vi "Binary_Array_To_Decimal_Array.vi"(10 "Nmbr_of_datapoints":dbl=128.0, 11 "Array In":u8[](array[numeric])) -> (0 "HEXVAL":string, 1 "nV":dbl, 2 "Loop count":dbl, 3 "Array Out":dbl[](array[numeric]))   [LabVIEW 2012]
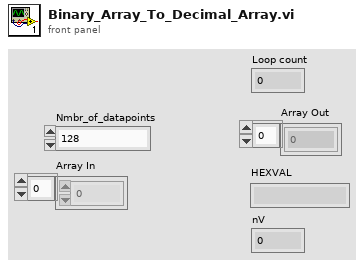
[diagram p1: front panel]
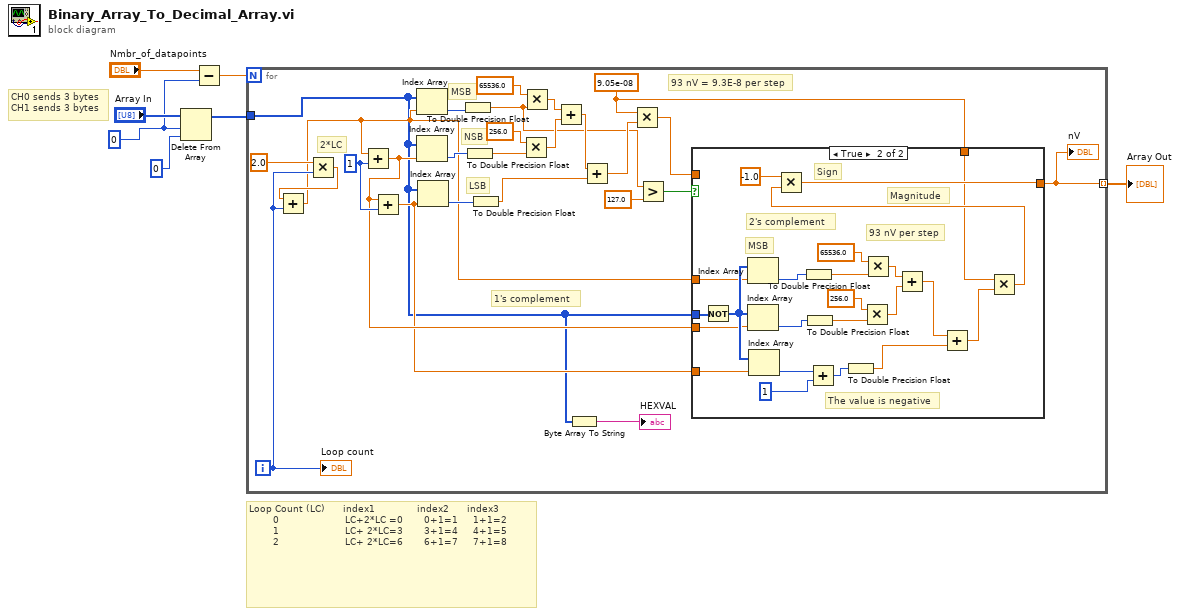
[diagram p0: block diagram]
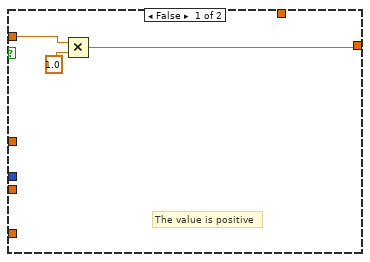
[diagram p2: hidden frame]
diagram:
  w3 = 0
  # "CH0 sends 3 bytes\nCH1 sends 3 bytes"
  # "Loop Count (LC)      index1              index2      index3      \n        0                      LC+2*LC =0       0+1=1     1+1=2\n        1                      LC+ 2*LC=3       3+1=4     4+1=5\n        2                      LC+ 2*LC=6       6+1=7     7+1=8"
  n1 = Delete From Array(array="Array In", length=w3, index=0) -> (array with subset deleted=w2:u8[])  [unwired: 1 out]
  n2 = Subtract(x="Nmbr_of_datapoints", y=w3) -> (x-y=w5:dbl)
  n3 = for {
    N: w5 -> [_]
    tunnel: w2 -> [w9]
    tunnel: [w8] -> w1 mode=indexing
    i -> [w15]
    w14 = 9.05e-08
    w25 = 1
    # "93 nV = 9.3E-8 per step"
    # "LSB"
    # "MSB"
    # "NSB"
    # "1's complement"
    # "2*LC"
    n4 = Multiply(x=2.0, y=w15) -> (x*y=w23:dbl)
    n5 = Add(x=w23, y=w15) -> (x+y=w13:dbl)
    n6 = Add(x=w13, y=w25) -> (x+y=w12:dbl)
    n7 = Add(x=w12, y=w25) -> (x+y=w11:dbl)
    n8 = Index Array(array=w9, index=w13) -> (element=w18:u8)
    n9 = Index Array(array=w9, index=w12) -> (element=w17:u8)
    n10 = Index Array(array=w9, index=w11) -> (element=w16:u8)
    n11 = To Double Precision Float(number=w18) -> (double precision float=w19:dbl)
    n12 = To Double Precision Float(number=w17) -> (double precision float=w31:dbl)
    n13 = To Double Precision Float(number=w16) -> (double precision float=w27:dbl)
    n14 = Multiply(x=256.0, y=w31) -> (x*y=w29:dbl)
    n15 = Multiply(x=65536.0, y=w19) -> (x*y=w33:dbl)
    n16 = Add(x=w33, y=w29) -> (x+y=w28:dbl)
    n17 = Byte Array To String(unsigned byte array=w9) -> (string=→"HEXVAL":string)
    n18 = Add(x=w28, y=w27) -> (x+y=w26:dbl)
    n19 = Multiply(x=w14, y=w26) -> (x*y=w22:dbl)
    n20 = Greater?(x=w19, y=127.0) -> (0:w21:bool)
    n21 = case shown="True" w21 {
      tunnel: [w36 w59] -> w8
      tunnel: w22 -> [w35 _]
      tunnel: w9 -> [_ w47]
      tunnel: w13 -> [_ w42]
      tunnel: w12 -> [_ w41]
      tunnel: w11 -> [_ w40]
      tunnel: w14 -> [_ w38]
      frame False {
        # "The value is positive"
        n22 = Multiply(x=w35, y=1.0) -> (x*y=w36:dbl)
      }
      frame True {
        # "The value is negative"
        # "93 nV per step"
        # "Magnitude"
        # "Sign"
        # "2's complement"
        # "MSB"
        n23 = Not(x=w47) -> (.not. x?=w46:u8[])
        n24 = Index Array(array=w46, index=w42) -> (element=w37:u8)
        n25 = Index Array(array=w46, index=w41) -> (element=w48:u8)
        n26 = Index Array(array=w46, index=w40) -> (element=w45:u8)
        n27 = To Double Precision Float(number=w37) -> (double precision float=w49:dbl)
        n28 = To Double Precision Float(number=w48) -> (double precision float=w55:dbl)
        n29 = Add(x=w45, y=1) -> (x+y=w43:i32)
        n30 = To Double Precision Float(number=w43) -> (double precision float=w51:dbl)
        n31 = Multiply(x=256.0, y=w55) -> (x*y=w53:dbl)
        n32 = Multiply(x=65536.0, y=w49) -> (x*y=w57:dbl)
        n33 = Add(x=w57, y=w53) -> (x+y=w52:dbl)
        n34 = Add(x=w52, y=w51) -> (x+y=w50:dbl)
        n35 = Multiply(x=w38, y=w50) -> (x*y=w39:dbl)
        n36 = Multiply(x=-1.0, y=w39) -> (x*y=w59:dbl)
      }
    }
    "nV" <- w8
    "Loop count" <- w15
  }
  "Array Out" <- w1
